vi "VIStep Configure UI.vi"(8 "error in (no error)":errorcluster, 10 "Project In":refnum<class "Project.lvclass">, 11 "ConfigureableObject in":refnum<class>) -> (0 "error out":errorcluster, 3 "ConfigureableObject out":refnum<class>)   [LabVIEW 2015, in "CallVIStep.lvclass"]
uses:
  CallVIStep.lvclass
  Project.lvclass
  UI_STATE.ctl
  Step.lvclass
  Editor/Editor.lvclass
panel:
  in  "Name":string
  in  "Stop If Fail":bool
  in  "Skip":bool
  in  "VI Path":path
  in  "Wait Until Completion":bool
  in  "Show Front Panel":bool
  in  "OutputPanelBtn":bool
  in  "InputPanelBtn":bool
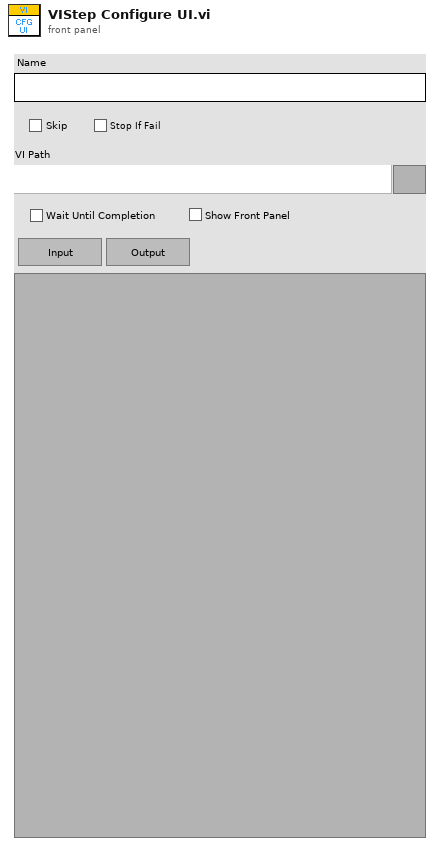
[diagram p1: front panel]
types:
  T1 = typedef "CallVIStep.lvclass/UI_STATE.ctl" = enum16{"UI_LOOP", "CHANGE_PANEL", "INIT", "END"}
  T2 = enum8{"Enabled", "Disabled", "Disabled and Grayed Out"}
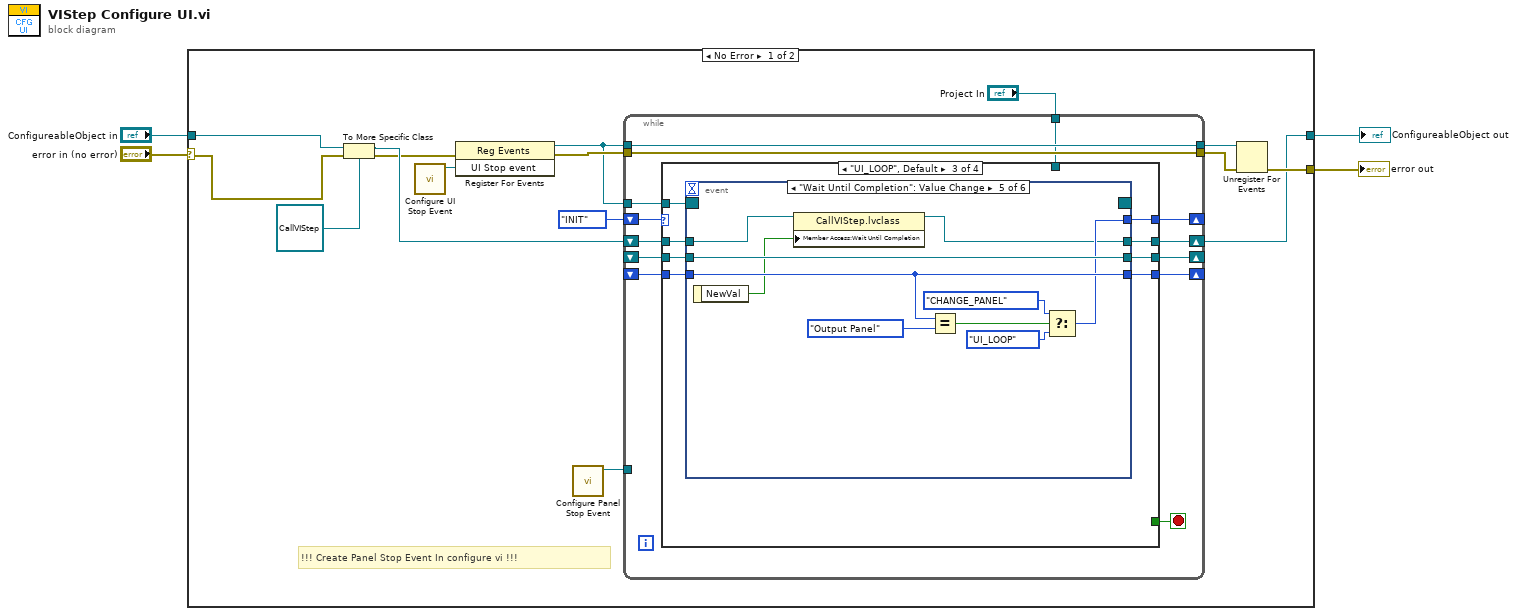
[diagram p0: block diagram]
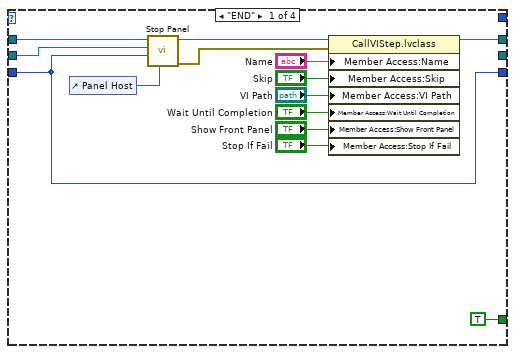
[diagram p2: hidden frame]
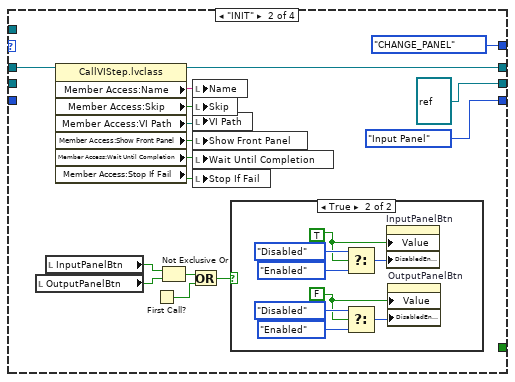
[diagram p3: hidden frame]
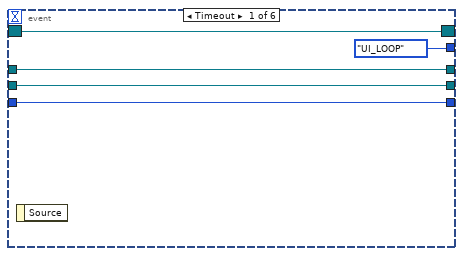
[diagram p5: hidden frame]
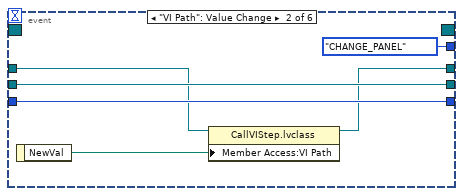
[diagram p6: hidden frame]
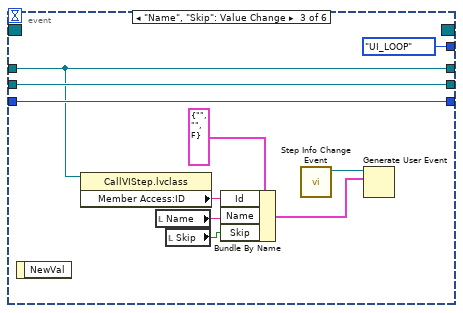
[diagram p7: hidden frame]
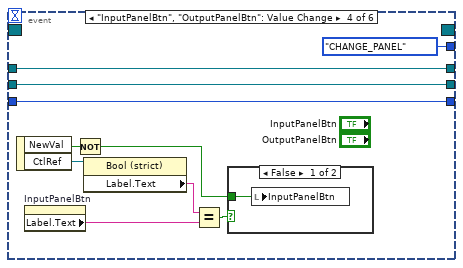
[diagram p8: hidden frame]
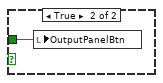
[diagram p9: hidden frame]
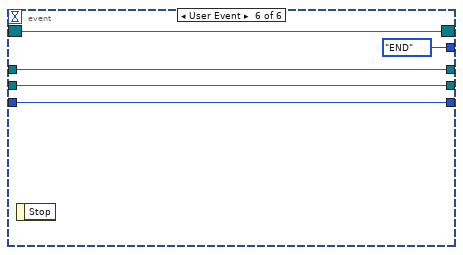
[diagram p10: hidden frame]
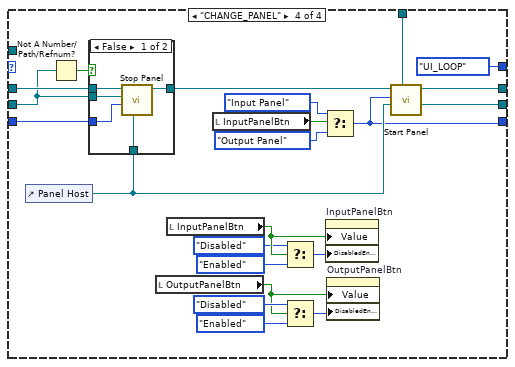
[diagram p11: hidden frame]
diagram:
  n1 = case shown="No Error" "error in (no error)" {
    selector: "error in (no error)" -> [w6 w156]
    tunnel: [w15 w156] -> w3
    tunnel: "ConfigureableObject in" -> [w19 w155]
    tunnel: [w14 w155] -> w1
    frame No Error {
      # "!!! Create Panel Stop Event In configure vi !!!"
      n2 = To More Specific Class(target class=refnum<class "CallVIStep.lvclass"> refnum ("CallVIStep.lvclass"), reference=w19, error in=w6) -> (specific class reference=w8:refnum<class "CallVIStep.lvclass">, error out=w7:errorcluster)
      n3 = call "Configure UI Stop Event.vi"() -> ("UI Stop event"=w9:refnum<user-event>)  [unwired: 11 in]
      n4 = register-events(error in=w7, w9) -> (reference out=w12:refnum<event-registration>, error out=w17:errorcluster)  [unwired: 1 in]
      n5 = call "Configure Panel Stop Event.vi"() -> ("Panel Stop event"=w10:refnum<user-event>)  [unwired: 11 in]
      n6 = while {
        tunnel: w12 -> [w32]
        tunnel: [w32] -> w18
        tunnel: w17 -> [w31]
        tunnel: [w31] -> w16
        shift-right: [w29] -> w14
        shift-left: w8 -> [w30]
        shift-right: [w27] -> _
        shift-left: UI_STATE."INIT" -> [w28]
        tunnel: w12 -> [w25]
        shift-right: [w24] -> _
        shift-left: _ -> [w23]
        shift-right: [w21] -> _
        shift-left: _ -> [w22]
        tunnel: w10 -> [_]
        tunnel: "Project In" -> [w20]
        stop <- w26 stop-if-true
        n7 = case shown="\"UI_LOOP\", Default" w28 {
          tunnel: w25 -> [_ _ w78 _]
          tunnel: w30 -> [w39 w62 w77 w147]
          tunnel: [w40 w55 w76 w142] -> w29
          tunnel: [_ UI_STATE."CHANGE_PANEL" w75 UI_STATE."UI_LOOP"] -> w27
          tunnel: [TRUE _ _ _] -> w26
          tunnel: [_ refnum<vi> refnum ("Panel VI out") w73 w140] -> w24
          tunnel: w23 -> [w37 _ w74 w145]
          tunnel: w22 -> [w34 _ w72 w146]
          tunnel: [w34 enum16{"Input Panel", "Output Panel"}."Input Panel" w71 w136] -> w21
          tunnel: w20 -> [_ _ _ w127]
          frame "END" {
            n8 = control-ref of="Panel Host"() -> (w35:refnum<vi>)
            n9 = call-dynamic "Stop Panel.vi"("Panel Host"=w35, "Panel"=w34, "Panel VI in"=w37, "CallVIStep in"=w39) -> ("error out"=w36:errorcluster, "CallVIStep out"=w38:refnum<class "CallVIStep.lvclass">)  [unwired: 6 in]
            n10 = property class="CallVIStep.lvclass"(reference=w38, error in=w36, "Member Access:Name"="Name", "Member Access:Skip"="Skip", "Member Access:VI Path"="VI Path", "Member Access:Wait Until Completion"="Wait Until Completion", "Member Access:Show Front Panel"="Show Front Panel", "Member Access:Stop If Fail"="Stop If Fail") -> (reference out=w40:refnum<class "CallVIStep.lvclass">)  [unwired: 1 out]
          }
          frame "INIT" {
            n11 = local read "OutputPanelBtn"() -> (w52:bool)
            n12 = local read "InputPanelBtn"() -> (w51:bool)
            n13 = property class="CallVIStep.lvclass"(reference=w62) -> (reference out=w55:refnum<class "CallVIStep.lvclass">, "Member Access:Name"=w61:string, "Member Access:Skip"=w60:bool, "Member Access:VI Path"=w59:path, "Member Access:Show Front Panel"=w58:bool, "Member Access:Wait Until Completion"=w57:bool, "Member Access:Stop If Fail"=w47:bool)  [unwired: 1 in, 1 out]
            n14 = First Call?() -> (First Call?: T/F=w49:bool)
            n15 = Not Exclusive Or(1:w52, 2:w51) -> (0:w50:bool)
            n16 = Or(x=w50, y=w49) -> (x .or. y?=w48:bool)
            n17 = local write "Name"(w61) -> ()
            n18 = local write "Skip"(w60) -> ()
            n19 = local write "VI Path"(w59) -> ()
            n20 = local write "Show Front Panel"(w58) -> ()
            n21 = local write "Wait Until Completion"(w57) -> ()
            n22 = local write "Stop If Fail"(w47) -> ()
            n23 = case shown="True" w48 {
              frame False {
              }
              frame True {
                w63 = FALSE
                w64 = TRUE
                n24 = Select(t=T2."Disabled" ("Disabled"), s=w64, f=T2."Enabled" ("Disabled")) -> (s? t:f=w69:T2)
                n25 = Select(t=T2."Disabled" ("Disabled"), s=w63, f=T2."Enabled" ("Disabled")) -> (s? t:f=w65:T2)
                n26 = property on="InputPanelBtn" class="Bool (strict)"("Value"=w64, "DisabledEnum"=w69) -> ()  [unwired: 2 in, 2 out]
                n27 = property on="OutputPanelBtn" class="Bool (strict)"("Value"=w63, "DisabledEnum"=w65) -> ()  [unwired: 2 in, 2 out]
              }
            }
          }
          frame "UI_LOOP", Default {
            n28 = event shown="[4] \"Wait Until Completion\": Value Change" {
              selector: w78 -> [w82 _ _ _ _ w125]
              dyn-events: [w82 _ _ _ _ w125] -> _
              timeout: _ -> [_ _ _ _ _ _]
              tunnel: w77 -> [w83 w86 w96 w109 w114 w126]
              tunnel: [w83 w84 w96 w109 w113 w126] -> w76
              tunnel: [UI_STATE."UI_LOOP" UI_STATE."CHANGE_PANEL" UI_STATE."UI_LOOP" UI_STATE."CHANGE_PANEL" w115 UI_STATE."END"] -> w75
              tunnel: [w81 w89 w99 w108 w121 w124] -> w73
              tunnel: w74 -> [w81 w89 w99 w108 w121 w124]
              tunnel: w72 -> [w80 w88 w98 w107 w119 w123]
              tunnel: [w80 w88 w98 w107 w119 w123] -> w71
              event Timeout {
                n29 = event-data() -> ()  [unwired: 1 in, 1 out]
              }
              event "VI Path": Value Change {
                n30 = event-data() -> ("NewVal"=w85:path)  [unwired: 1 in]
                n31 = property class="CallVIStep.lvclass"(reference=w86, "Member Access:VI Path"=w85) -> (reference out=w84:refnum<class "CallVIStep.lvclass">)  [unwired: 1 in, 1 out]
              }
              event "Name", "Skip": Value Change {
                n32 = event-data() -> ()  [unwired: 1 in, 1 out]
                n33 = property class="CallVIStep.lvclass"(reference=w96) -> ("Member Access:ID"=w94:string)  [unwired: 1 in, 2 out]
                n34 = local read "Name"() -> (w92:string)
                n35 = local read "Skip"() -> (w91:bool)
                n36 = Bundle By Name(cluster=cluster{"Id":string, "Name":string, "Skip":bool} {"Id"="", "Name"="", "Skip"=FALSE} ("Step Info"), "Id"=w94, "Name"=w92, "Skip"=w91) -> (w90:cluster{"Id":string, "Name":string, "Skip":bool})
                n37 = call "Step Info Change Event.vi"() -> ("Step Info Change Event"=w95:refnum<user-event>)  [unwired: 11 in]
                n38 = Generate User Event(user event=w95, event data cluster=w90) -> ()  [unwired: 2 in, 2 out]
              }
              event "InputPanelBtn", "OutputPanelBtn": Value Change {
                n39 = event-data() -> ("NewVal"=w102:bool, "CtlRef"=w105:refnum<vi>)  [unwired: 1 in]
                n40 = property on="InputPanelBtn" class="Bool (strict)"() -> ("Label.Text"=w100:string)  [unwired: 2 in, 2 out]
                n41 = Not(x=w102) -> (.not. x?=w101:bool)
                n42 = property class="Bool (strict)"(reference=w105) -> ("Label.Text"=w104:string)  [unwired: 1 in, 2 out]
                n43 = Equal?(x=w104, y=w100) -> (x = y?=w103:bool)
                n44 = case shown="False" w103 {
                  tunnel: w101 -> [w110 w111]
                  frame False {
                    n45 = local write "InputPanelBtn"(w110) -> ()
                  }
                  frame True {
                    n46 = local write "OutputPanelBtn"(w111) -> ()
                  }
                }
              }
              event "Wait Until Completion": Value Change {
                n47 = event-data() -> ("NewVal"=w112:bool)  [unwired: 1 in]
                n48 = property class="CallVIStep.lvclass"(reference=w114, "Member Access:Wait Until Completion"=w112) -> (reference out=w113:refnum<class "CallVIStep.lvclass">)  [unwired: 1 in, 1 out]
                n49 = Equal?(x=w119, y=enum16{"Input Panel", "Output Panel"}."Output Panel") -> (x = y?=w118:bool)
                n50 = Select(t=UI_STATE."CHANGE_PANEL", s=w118, f=UI_STATE."UI_LOOP") -> (s? t:f=w115:T1)
              }
              event User Event {
                n51 = event-data() -> ()  [unwired: 1 in, 1 out]
              }
            }
          }
          frame "CHANGE_PANEL" {
            n52 = control-ref of="Panel Host"() -> (w141:refnum<vi>)
            n53 = Not A Number/Path/Refnum?(number/path/refnum=w145) -> (NaN/Path/Refnum?=w144:bool)
            n54 = case shown="False" w144 {
              tunnel: w147 -> [w153 w154]
              tunnel: w146 -> [w152 _]
              tunnel: [w151 w154] -> w143
              tunnel: w145 -> [w150 _]
              tunnel: w141 -> [w149 _]
              frame False {
                n55 = call-dynamic "Stop Panel.vi"("Panel Host"=w149, "Panel"=w152, "Panel VI in"=w150, "CallVIStep in"=w153) -> ("CallVIStep out"=w151:refnum<class "CallVIStep.lvclass">)  [unwired: 6 in, 1 out]
              }
              frame True {
              }
            }
            n56 = local read "OutputPanelBtn"() -> (w128:bool)
            n57 = local read "InputPanelBtn"() -> (w133:bool)
            n58 = local read "InputPanelBtn"() -> (w139:bool)
            n59 = Select(t=T2."Disabled" ("Disabled"), s=w133, f=T2."Enabled" ("Disabled")) -> (s? t:f=w134:T2)
            n60 = Select(t=T2."Disabled" ("Disabled"), s=w128, f=T2."Enabled" ("Disabled")) -> (s? t:f=w129:T2)
            n61 = Select(t=enum16{"Input Panel", "Output Panel"}."Input Panel", s=w139, f=enum16{"Input Panel", "Output Panel"}."Output Panel") -> (s? t:f=w136:enum16{"Input Panel", "Output Panel"})
            n62 = property on="InputPanelBtn" class="Bool (strict)"("Value"=w133, "DisabledEnum"=w134) -> ()  [unwired: 2 in, 2 out]
            n63 = property on="OutputPanelBtn" class="Bool (strict)"("Value"=w128, "DisabledEnum"=w129) -> ()  [unwired: 2 in, 2 out]
            n64 = call-dynamic "Start Panel.vi"("Project In"=w127, "Panel Host"=w141, "Panel"=w136, "CallVIStep in"=w143) -> ("Panel VI out"=w140:refnum<vi>, "CallVIStep out"=w142:refnum<class "CallVIStep.lvclass">)  [unwired: 5 in, 1 out]
          }
        }
      }
      n65 = Unregister For Events(event registration refnum=w18, error in=w16) -> (error out=w15:errorcluster)
    }
    frame Error {
    }
  }
  "error out" <- w3
  "ConfigureableObject out" <- w1
